vi "supressStraylight.vi"(6 "DestSpectrum":dbl[](array[numeric]), 7 "Device":i32, 8 "error in (no error)":errorcluster, 9 "SrcSpectrum":dbl[](array[numeric]), 10 "Multifactor":sgl, 11 "SEDSpectrometer in":refnum<class "SEDSpectrometer.lvclass">) -> (0 "error out":errorcluster, 1 "a_pSrcSpectrum":dbl[](array[numeric]), 2 "Output Value":i32, 3 "SEDSpectrometer out":refnum<class "SEDSpectrometer.lvclass">)   [LabVIEW 2016, in "SEDSpectrometer.lvclass"]
uses:
  SEDSpectrometer.lvclass
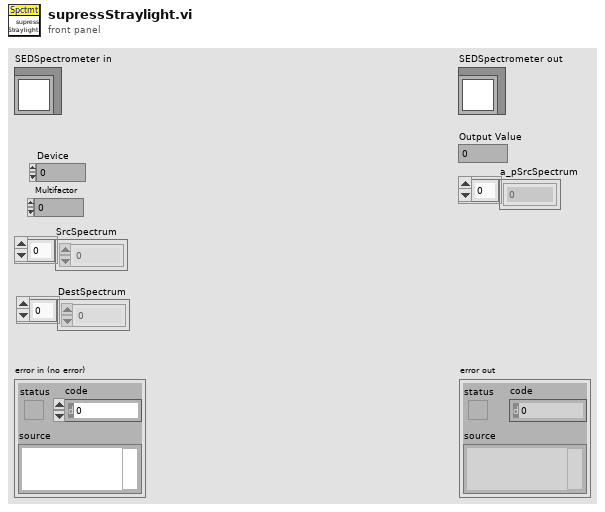
[diagram p1: front panel]
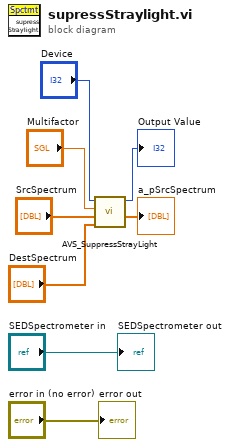
[diagram p0: block diagram]
diagram:
  n1 = call "AVS_SuppressStrayLight.vi"("a_pDestSpectrum"="DestSpectrum", "a_pSrcSpectrum"="SrcSpectrum", "a_Multifactor"="Multifactor", "a_hDevice"="Device") -> ("a_pSrcSpectrum"=→"a_pSrcSpectrum":dbl[], "Output Value"=→"Output Value":i32)  [unwired: 1 in, 1 out]
  "error out" <- "error in (no error)"
  "SEDSpectrometer out" <- "SEDSpectrometer in"
